vi "ActivateFirstePages.vi"(8 "Error In":errorcluster, 11 "TabCtl Refnum":refnum<vi>) -> (0 "Error Out":errorcluster)   [LabVIEW 2013, in "main.lvlib"]
uses:
  main.lvlib
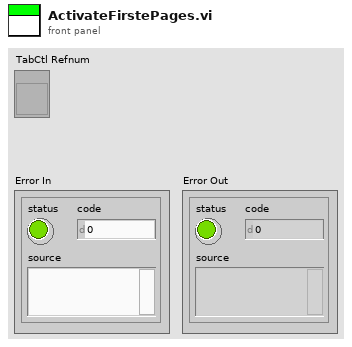
[diagram p1: front panel]
types:
  T1 = enum32{"Page Enabled", "Page Disabled", "Page Disabled & Grayed"}
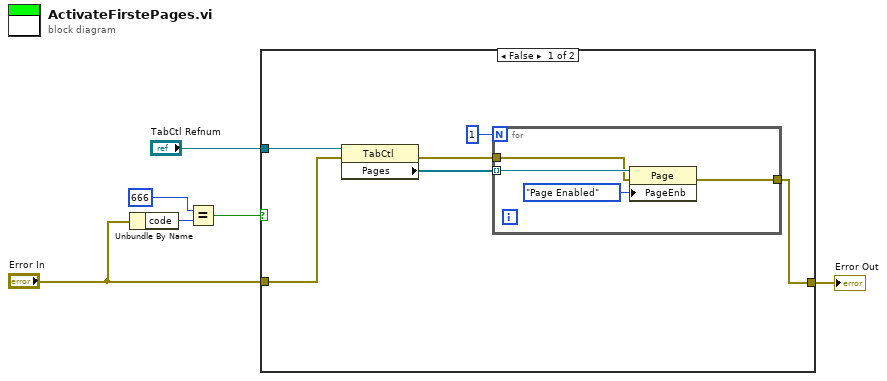
[diagram p0: block diagram]
diagram:
  n1 = Unbundle By Name("Error In") -> ("code"=w6:i32)
  n2 = Equal?(x=666, y=w6) -> (x = y?=w4:bool)
  n3 = case shown="False" w4 {
    tunnel: "Error In" -> [w10 w17]
    tunnel: [w8 w17] -> w2
    tunnel: "TabCtl Refnum" -> [w7 _]
    frame False {
      n4 = property class="TabCtl"(reference=w7, error in=w10) -> (error out=w9:errorcluster, "Pages"=w12:refnum<vi>[])  [unwired: 1 out]
      n5 = for {
        N: 1 -> [_]
        tunnel: w12 -> [w16] mode=indexing
        tunnel: w9 -> [w14]
        tunnel: [w13] -> w8
        n6 = property class="Page"(reference=w16, error in=w14, "PageEnb"=T1."Page Enabled" ("Page Enabled State")) -> (error out=w13:errorcluster)  [unwired: 1 out]
      }
    }
    frame True {
    }
  }
  "Error Out" <- w2
